vi "SatoPrinter.vi"() -> ()   [LabVIEW 2017]
uses:
  <vilib>/Utility/NIReport.llb/NI_ReportGenerationCore.lvlib
panel:
  in  "Print":bool
  out "PrinterName":string
  in  "SelectPrinter":u16(ring) items=["SATO CL4NX 203dpi", "Send To OneNote 2016", "OneNote", "Microsoft XPS Document Writer", "Microsoft Print to PDF", "Fax", "CutePDF Writer", "Adobe PDF"]
  in  "stop":bool
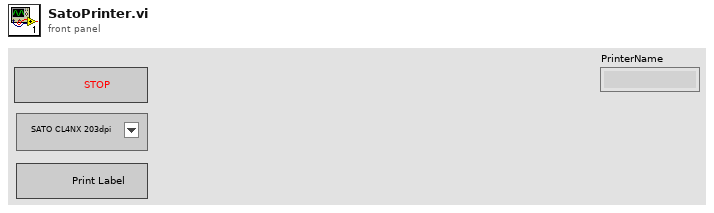
[diagram p1: front panel]
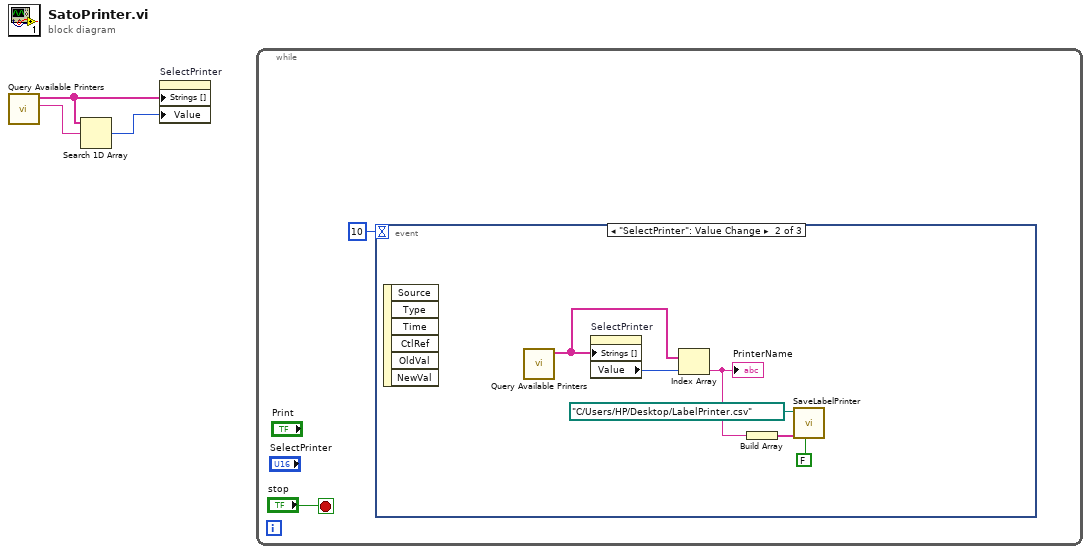
[diagram p0: block diagram]
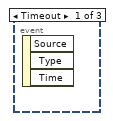
[diagram p2: hidden frame]
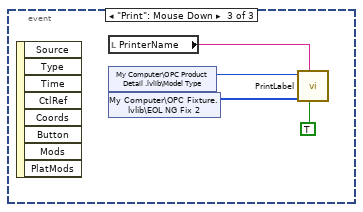
[diagram p3: hidden frame]
diagram:
  n1 = call <vilib>:"Query Available Printers.vi"() -> ("default printer"=w3:string, "system configured printers"=w2:string[])  [unwired: 9 in, 1 out]
  n2 = Search 1D Array(1D array=w2, element=w3) -> (index of element=w1:i32)  [unwired: 1 in]
  n3 = property on="SelectPrinter" class="Ring (strict)"("Strings []"=w2, "Value"=w1) -> ()  [unwired: 2 in, 2 out]
  n4 = while {
    stop <- "stop" stop-if-true
    n5 = event shown="[1] \"SelectPrinter\": Value Change" {
      selector: _ -> [_ _ _]
      dyn-events: _ -> [_ _ _]
      timeout: 10 -> [_ _ _]
      event Timeout {
        n6 = event-data() -> ()  [unwired: 1 in, 3 out]
      }
      event "SelectPrinter": Value Change {
        n7 = event-data() -> ()  [unwired: 1 in, 6 out]
        n8 = call <vilib>:"Query Available Printers.vi"() -> ("system configured printers"=w10:string[])  [unwired: 9 in, 2 out]
        n9 = property on="SelectPrinter" class="Ring (strict)"("Strings []"=w10) -> ("Value"=w11:u16)  [unwired: 2 in, 2 out]
        n10 = Index Array(array=w10, index=w11) -> (element=w8:string)
        "PrinterName" <- w8
        n11 = Build Array(w8) -> (w7:string[])
        n12 = call "SaveLabelPrinter.vi"("En Pop up"=FALSE, "LabelPrinterName"=w7, "Save Path"=path "C:/Users/HP/Desktop/LabelPrinter.csv") -> ()  [unwired: 8 in, 1 out]
      }
      event "Print": Mouse Down {
        n13 = event-data() -> ()  [unwired: 1 in, 8 out]
        n14 = local read "PrinterName"() -> (w13:string)
        n15 = shared-variable "My Computer\\OPC Product Detail .lvlib\\Model Type"() -> (w15:u16)  [unwired: 1 in, 1 out]
        n16 = shared-variable "My Computer\\OPC Fixture.lvlib\\EOL NG Fix 2"() -> (w14:u16[])  [unwired: 1 in, 1 out]
        n17 = call "PrintLabel.vi"("Print"=TRUE, "printer name (default)"=w13, "Fixture_Data"=w14, "OPC_Model Type"=w15) -> ()  [unwired: 8 in]
      }
    }
  }
